vi "2_avg_formula.vi"(1 "B":dbl, 2 "A":dbl) -> (0 "OP":dbl)   [LabVIEW 2026]
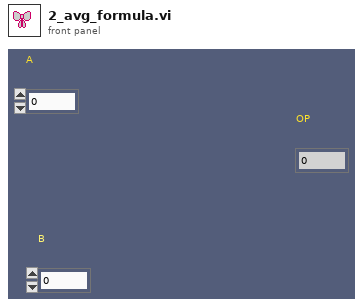
[diagram p1: front panel]
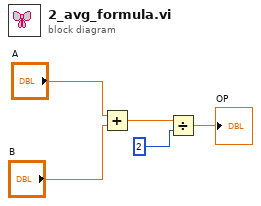
[diagram p0: block diagram]
diagram:
  n1 = Add(x="A", y="B") -> (x+y=w3:dbl)
  n2 = Divide(x=w3, y=2) -> (x/y=→"OP":dbl)
